vi "draw_point_sprite.vi"(7 "Transformation":sgl[][](array[numeric]), 8 "Enum":T1(ring)=enum."EmptySquare", 9 "quadsize (4)":sgl=2.0, 10 "Color Array":T2[](array[typedef]), 11 "Vertex Array":T3[](array[typedef])) -> (3 "Scene:New Object":refnum<vi>)   [LabVIEW 2020, in "3DPC_SurfacePlot.xctl"]
uses:
  <vilib>/Native 3D Graph/xcontrol/3DPC_SurfacePlot.xctl
  <vilib>/Utility/miscctls.llb/LV3DPointTypeDef.ctl
  <vilib>/Utility/miscctls.llb/LVRGBAColorTypeDef.ctl
  <vilib>/Utility/miscctls.llb/LVTextureCoordinateArrayTypeDef.ctl
  <vilib>/picture/picture.llb/imagedata.ctl
  <vilib>/picture/3D Picture Control/Object/Create Object (name).vi
  <vilib>/picture/3D Picture Control/NI_3D Picture Control.lvlib
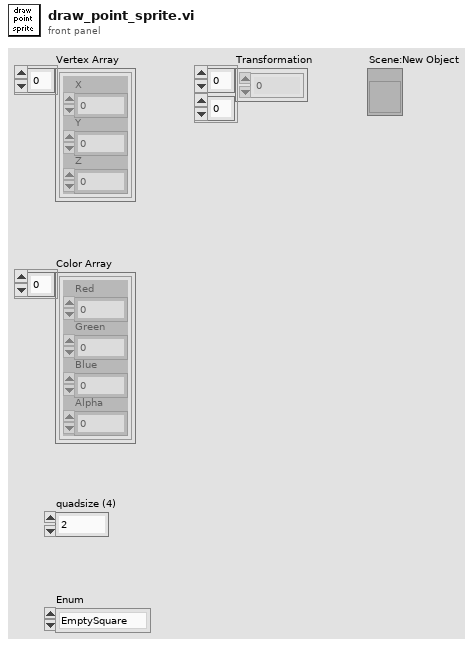
[diagram p1: front panel]
types:
  T1 = enum16{"Point", "EmptySquare", "Asterisk", "Diamond", "EmptyCircle", "Circle", "X"}
  T2 = typedef "LVRGBAColorTypeDef.ctl" = cluster{"Red":sgl, "Green":sgl, "Blue":sgl, "Alpha":sgl}
  T3 = typedef "LV3DPointTypeDef.ctl" = cluster{"X":sgl, "Y":sgl, "Z":sgl}
  T4 = enum16{"Normal Bin", "Opaque Bin", "Transparent Bin"}
  T5 = enum16{"Overall", "Per Primitive", "Per Vertex", "Binding Off"}
  T6 = typedef "LVTextureCoordinateArrayTypeDef.ctl" = cluster{"S":sgl, "T":sgl}[]
  T7 = enum16{"Points", "Lines", "Line Strip", "Line Loop", "Triangles", "Triangle Strip", "Triangle Fan", "Quads", "Quad Strip", "Polygon"}
  T8 = enum16{"As a Decal", "With Modulation", "With Blending", "As a replacement"}
  T9 = typedef "imagedata.ctl" = cluster{"image type":i32, "image depth":i32, "image":u8[], "mask":u8[], "colors":u32[], "Rectangle":cluster{"left":i16, "top":i16, "right":i16, "bottom":i16}}
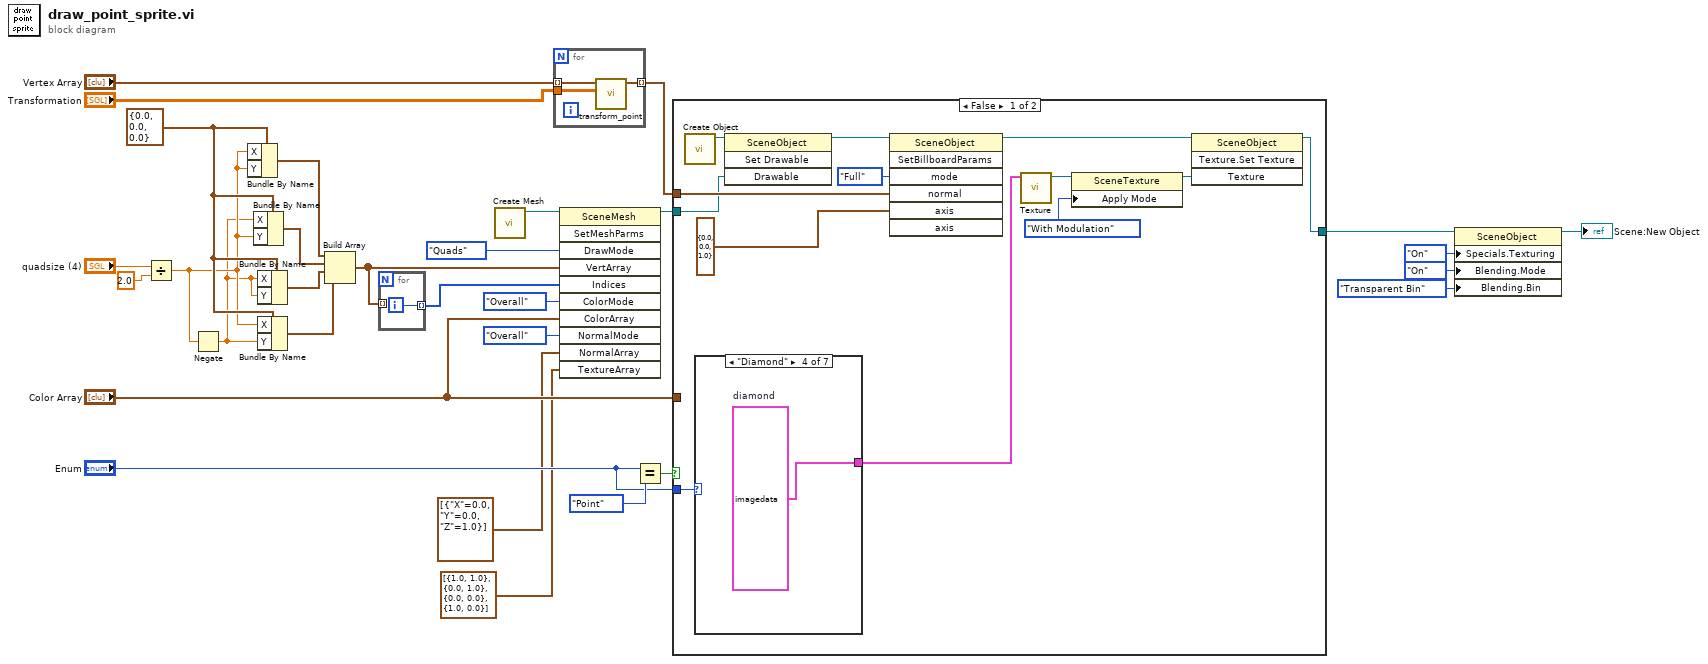
[diagram p0: block diagram]
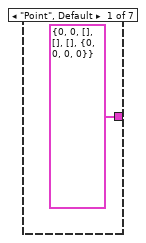
[diagram p2: hidden frame]
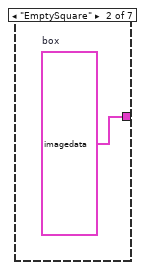
[diagram p3: hidden frame]
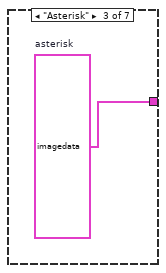
[diagram p4: hidden frame]
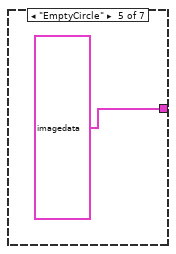
[diagram p5: hidden frame]
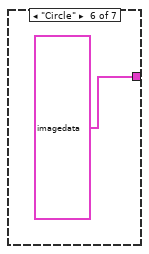
[diagram p6: hidden frame]
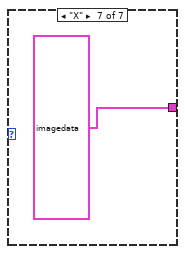
[diagram p7: hidden frame]
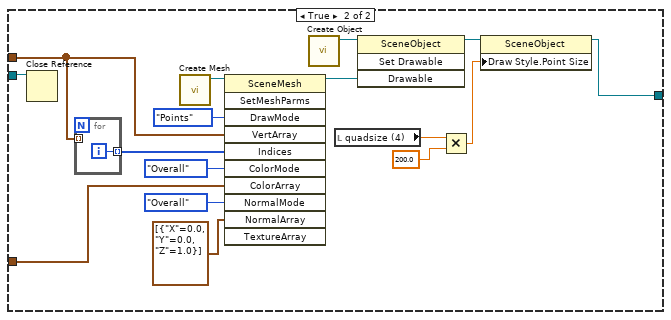
[diagram p8: hidden frame]
diagram:
  w20 = T3 {"X"=0.0, "Y"=0.0, "Z"=0.0} ("3D Point")
  n1 = Divide(x="quadsize (4)", y=sgl 2.0) -> (x/y=w16:sgl)
  n2 = Negate(x=w16) -> (-x=w15:sgl)
  n3 = Bundle By Name(cluster=w20, "X"=w16, "Y"=w16) -> (w14:T3)
  n4 = Bundle By Name(cluster=w20, "X"=w15, "Y"=w16) -> (w13:T3)
  n5 = Bundle By Name(cluster=w20, "X"=w15, "Y"=w15) -> (w12:T3)
  n6 = Bundle By Name(cluster=w20, "X"=w16, "Y"=w15) -> (w11:T3)
  n7 = Build Array(w14, w13, w12, w11) -> (w10:T3[])
  n8 = for {
    tunnel: [w31] -> w26 mode=indexing
    tunnel: w10 -> [_] mode=indexing
    i -> [w31]
  }
  n9 = call <vilib>:"Create Mesh.vi"() -> ("New Mesh Refnum"=w27:refnum<vi>)  [unwired: 1 in, 10 out]
  n10 = for {
    tunnel: "Vertex Array" -> [w33] mode=indexing
    tunnel: "Transformation" -> [w34]
    tunnel: [w32] -> w6 mode=indexing
    n11 = call <vilib>:"transform_point.vi"("Transformation"=w34, "3D Point"=w33) -> ("output cluster"=w32:T3)  [unwired: 9 out]
  }
  n12 = invoke class="SceneMesh" method="SetMeshParms"(reference=w27, "DrawMode"=T7."Quads" ("Draw Mode"), "VertArray"=w10, "Indices"=w26, "ColorMode"=T5."Overall" ("Color Binding Mode"), "ColorArray"="Color Array", "NormalMode"=T5."Overall" ("Normal Binding Mode"), "NormalArray"=T3[] [{"X"=0.0, "Y"=0.0, "Z"=1.0}] ("Normal Array"), "TextureArray"=T6 [{"S"=1.0, "T"=1.0}, {"S"=0.0, "T"=1.0}, {"S"=0.0, "T"=0.0}, {"S"=1.0, "T"=0.0}] ("Texture Coordinate Array")) -> (reference out=w19:refnum<vi>)  [unwired: 2 in, 10 out]
  n13 = Equal?(x="Enum", y=T1."Point") -> (x = y?=w23:bool)
  n14 = case shown="False" w23 {
    tunnel: [w42 w64] -> w25
    tunnel: "Enum" -> [w44 _]
    tunnel: w6 -> [w41 w55]
    tunnel: w19 -> [w38 w58]
    tunnel: "Color Array" -> [_ w68]
    frame False {
      n15 = call-poly <vilib>:"Create Object.vi"() -> ("Scene:New Object"=w39:refnum<vi>)  [unwired: 10 in, 1 out]
      n16 = case shown="\"Diamond\"" w44 {
        tunnel: [T9 {"image type"=0, "image depth"=0, "image"=[], "mask"=[], "colors"=[], "Rectangle"={"left"=0, "top"=0, "right"=0, "bottom"=0}} ("output cluster") w49 w50 w51 T9 {"image type"=0, "image depth"=32, "image"=array[4096 elements], "mask"=[], "colors"=[], "Rectangle"={"left"=0, "top"=0, "right"=32, "bottom"=32}} ("output cluster") T9 {"image type"=0, "image depth"=32, "image"=array[4096 elements], "mask"=[], "colors"=[], "Rectangle"={"left"=0, "top"=0, "right"=32, "bottom"=32}} ("output cluster") T9 {"image type"=0, "image depth"=32, "image"=array[4096 elements], "mask"=[], "colors"=[], "Rectangle"={"left"=0, "top"=0, "right"=32, "bottom"=32}} ("output cluster")] -> w47
        frame "Point", Default {
        }
        frame "EmptySquare" {
          w49 = T9 {"image type"=0, "image depth"=32, "image"=array[4096 elements], "mask"=[], "colors"=[], "Rectangle"={"left"=0, "top"=0, "right"=32, "bottom"=32}}  # box
        }
        frame "Asterisk" {
          w50 = T9 {"image type"=0, "image depth"=32, "image"=array[4096 elements], "mask"=[], "colors"=[], "Rectangle"={"left"=0, "top"=0, "right"=32, "bottom"=32}}  # asterisk
        }
        frame "Diamond" {
          w51 = T9 {"image type"=0, "image depth"=32, "image"=array[4096 elements], "mask"=[], "colors"=[], "Rectangle"={"left"=0, "top"=0, "right"=32, "bottom"=32}}  # diamond
        }
        frame "EmptyCircle" {
        }
        frame "Circle" {
        }
        frame "X" {
        }
      }
      n17 = invoke class="SceneObject" method="Set Drawable"(reference=w39, "Drawable"=w38) -> (reference out=w37:refnum<vi>)  [unwired: 2 in, 3 out]
      n18 = invoke class="SceneObject" method="SetBillboardParams"(reference=w37, "mode"=enum16{"No Billboarding", "Axial", "Full"}."Full", "normal"=w41, "axis"=T3 {"X"=0.0, "Y"=0.0, "Z"=1.0} ("normal")) -> (reference out=w43:refnum<vi>)  [unwired: 3 in, 6 out]
      n19 = call <vilib>:"Texture.vi"("Image"=w47) -> ("New Texture Refnum"=w35:refnum<vi>)  [unwired: 1 in, 9 out]
      n20 = property class="SceneTexture"(reference=w35, "Apply Mode"=T8."With Modulation") -> (reference out=w45:refnum<vi>)  [unwired: 1 in, 1 out]
      n21 = invoke class="SceneObject" method="Texture.Set Texture"(reference=w43, "Texture"=w45) -> (reference out=w42:refnum<vi>)  [unwired: 2 in, 3 out]
    }
    frame True {
      n22 = Close Reference(reference=w58) -> ()  [unwired: 1 in, 1 out]
      n23 = for {
        tunnel: [w71] -> w69 mode=indexing
        tunnel: w55 -> [_] mode=indexing
        i -> [w71]
      }
      n24 = call <vilib>:"Create Mesh.vi"() -> ("New Mesh Refnum"=w62:refnum<vi>)  [unwired: 1 in, 10 out]
      n25 = invoke class="SceneMesh" method="SetMeshParms"(reference=w62, "DrawMode"=T7."Points" ("Draw Mode"), "VertArray"=w55, "Indices"=w69, "ColorMode"=T5."Overall" ("Normal Binding Mode"), "ColorArray"=w68, "NormalMode"=T5."Overall" ("Normal Binding Mode"), "NormalArray"=T3[] [{"X"=0.0, "Y"=0.0, "Z"=1.0}] ("Normal Array")) -> (reference out=w67:refnum<vi>)  [unwired: 3 in, 10 out]
      n26 = call-poly <vilib>:"Create Object.vi"() -> ("Scene:New Object"=w70:refnum<vi>)  [unwired: 10 in, 1 out]
      n27 = local read "quadsize (4)"() -> (w61:sgl)
      n28 = invoke class="SceneObject" method="Set Drawable"(reference=w70, "Drawable"=w67) -> (reference out=w65:refnum<vi>)  [unwired: 2 in, 3 out]
      n29 = Multiply(x=w61, y=sgl 200.0) -> (x*y=w59:sgl)
      n30 = property class="SceneObject"(reference=w65, "Draw Style.Point Size"=w59) -> (reference out=w64:refnum<vi>)  [unwired: 1 in, 1 out]
    }
  }
  n31 = property class="SceneObject"(reference=w25, "Specials.Texturing"=enum16{"Inherit Value", "Off", "On"}."On" ("Specials:Texturing"), "Blending.Mode"=enum16{"Inherit Value", "Off", "On"}."On" ("Blending:Mode"), "Blending.Bin"=T4."Transparent Bin" ("Blending:Bin")) -> (reference out=→"Scene:New Object":refnum<vi>)  [unwired: 1 in, 1 out]
